vi "test Container Lease.vi"(8 "error in (no error)":errorcluster, 11 "TestCase in":refnum<class "Test_Blob.lvclass">) -> (0 "error out":errorcluster, 3 "TestCase out":refnum<class "Test_Blob.lvclass">)   [LabVIEW 2015, in "Test_Blob.lvclass"]
uses:
  Test_Blob.lvclass
  Global Parameters.vi
  Core/Session/Session.lvclass
  Blob Storage/NI_Azure_Blob.lvlib
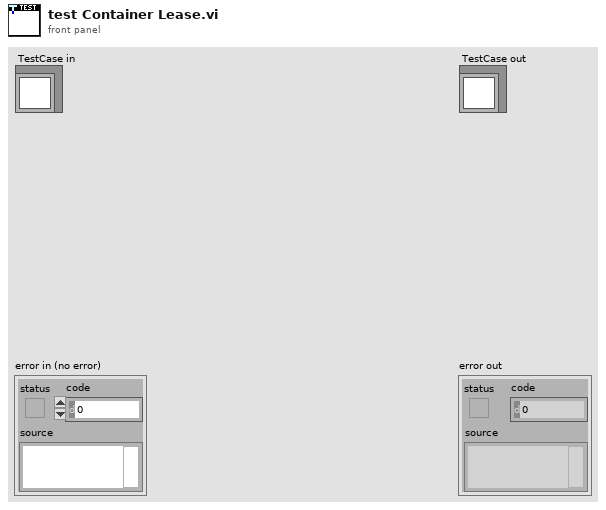
[diagram p1: front panel]
types:
  T1 = typedef "NI_Azure_Core.lvlib/Session.lvclass/Azure Credentials.ctl" = cluster{"Storage Account Name":string, "Access Key":string}
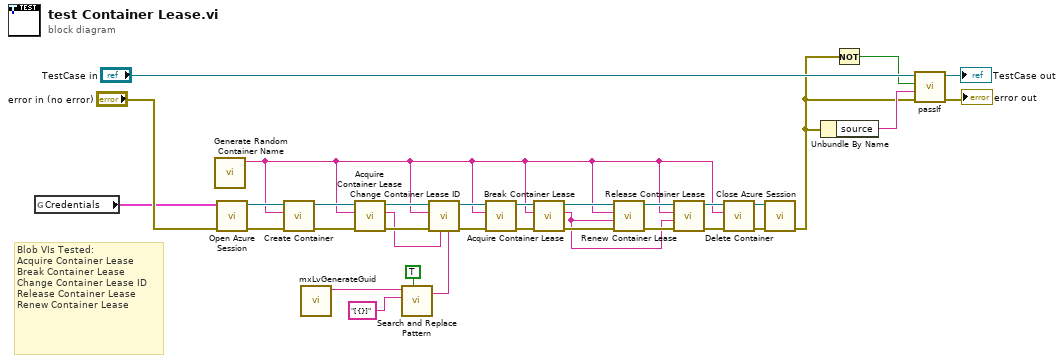
[diagram p0: block diagram]
diagram:
  # "Blob VIs Tested:\nAcquire Container Lease\nBreak Container Lease\nChange Container Lease ID\nRelease Container Lease\nRenew Container Lease"
  n1 = global read "Global Parameters.vi" "Credentials"() -> (w25:T1)
  n2 = call "Generate Random Container Name.vi"() -> ("Random Container Name"=w4:string)  [unwired: 11 in]
  n3 = call "Open Azure Session.vi"("error in (no error)"="error in (no error)", "Credentials"=w25) -> ("error out"=w26:errorcluster, "Azure Session"=w23:refnum<class "Session.lvclass">)  [unwired: 8 in]
  n4 = call "Create Container.vi"("error in (no error)"=w26, "Container"=w4, "Azure Session in"=w23) -> ("error out"=w29:errorcluster, "Azure Session out"=w28:refnum<class "Session.lvclass">)  [unwired: 7 in]
  n5 = call <resource>:"mxLvGenerateGuid.vi"() -> ("Value"=w16:string)  [unwired: 10 in, 1 out]
  n6 = call "Acquire Container Lease.vi"("error in (no error)"=w29, "Container"=w4, "Azure Session in"=w28) -> ("error out"=w21:errorcluster, "Lease ID"=w1:string, "Azure Session out"=w19:refnum<class "Session.lvclass">)  [unwired: 6 in]
  n7 = call <vilib>:"Search and Replace Pattern.vi"("string"=w16, "regular expression (\"\")"="[{}]" ("regular expression (\"\")"), "replace all? (F)"=TRUE) -> ("result string"=w2:string)  [unwired: 2 in, 1 out]
  n8 = call "Change Container Lease ID.vi"("Proposed Lease ID"=w2, "Current Lease ID"=w1, "error in (no error)"=w21, "Container"=w4, "Azure Session in"=w19) -> ("error out"=w20:errorcluster, "Azure Session out"=w12:refnum<class "Session.lvclass">)  [unwired: 5 in]
  n9 = call "Break Container Lease.vi"("error in (no error)"=w20, "Container"=w4, "Azure Session in"=w12) -> ("error out"=w13:errorcluster, "Azure Session out"=w6:refnum<class "Session.lvclass">)  [unwired: 7 in]
  n10 = call "Acquire Container Lease.vi"("error in (no error)"=w13, "Container"=w4, "Azure Session in"=w6) -> ("error out"=w7:errorcluster, "Lease ID"=w3:string, "Azure Session out"=w5:refnum<class "Session.lvclass">)  [unwired: 6 in]
  n11 = call "Renew Container Lease.vi"("error in (no error)"=w7, "Lease ID"=w3, "Container"=w4, "Azure Session in"=w5) -> ("error out"=w11:errorcluster, "Azure Session out"=w9:refnum<class "Session.lvclass">)  [unwired: 6 in]
  n12 = call "Release Container Lease.vi"("error in (no error)"=w11, "Lease ID"=w3, "Container"=w4, "Azure Session in"=w9) -> ("error out"=w10:errorcluster, "Azure Session out"=w8:refnum<class "Session.lvclass">)  [unwired: 6 in]
  n13 = call "Delete Container.vi"("error in (no error)"=w10, "Container"=w4, "Azure Session in"=w8) -> ("error out"=w24:errorcluster, "Azure Session out"=w22:refnum<class "Session.lvclass">)  [unwired: 7 in]
  n14 = call "Close Azure Session.vi"("error in (no error)"=w24, "Azure Session"=w22) -> ("error out"=w18:errorcluster)  [unwired: 9 in]
  n15 = Unbundle By Name(w18) -> ("source"=w30:string)
  n16 = Not(x=w18) -> (.not. x?=w17:bool)
  n17 = call-dynamic "passIf.vi"("error in (no error)"=w18, "message (\"\")"=w30, "pass"=w17, "TestCase in"="TestCase in") -> ("error out"=→"error out":errorcluster, "TestCase out"=→"TestCase out":refnum<class "Test_Blob.lvclass">)  [unwired: 6 in]
